vi "Finish.vi"   [LabVIEW 2013]
doc: "This VI is called just before exiting. It is expected to close I/O refnum, save collected data, etc."
uses:
  <vilib>/Rock Robotics/WPI/Joystick/WPI_JoystickGetSetRefNum.vi
  <vilib>/Rock Robotics/WPI/RobotDrive/WPI_RobotDriveGetSetRefNum.vi
types:
  T1 = typedef "WPI_JoystickDevRef.ctl" = cluster{"Device":T2}
  T2 = typedef "WPI_JoystickDeviceEnum.ctl" = enum16{"USB 1", "USB 2", "USB 3", "USB 4", "Kinect 1", "Kinect 2"}
  T3 = typedef "WPI_RobotDriveDevRef.ctl" = cluster{"DevStatus":errorcluster, "Motors[]":T4[], "Square Inputs":bool, "Max Output":dbl, "Isochronous":bool}
  T4 = typedef "WPI_MotorControlDeviceRef.ctl" = cluster{"DeviceStatus":errorcluster, "Type":enum16{"PWM", "CAN"}, "PWM":cluster{"Digital Module":T5, "PWM Channel":T6, "DeadBand":T7}, "CAN":cluster{"Device Number":u8, "Control Mode":T8, "Semaphore":T9, "Max Vout":dbl}, "Invert":bool, "TransformRef":T10, "InvTransformRef":T10}
  T5 = typedef "FPGA_TypedefDigitalModule.ctl" = enum16{"Digital Module 1", "Digital Module 2"}
  T6 = typedef "FPGA_DIOPWMChannel.ctl" = enum8{"PWM 1", "PWM 2", "PWM 3", "PWM 4", "PWM 5", "PWM 6", "PWM 7", "PWM 8", "PWM 9", "PWM 10", "Invalid"}
  T7 = typedef "WPI_PWMDeadband.ctl" = cluster{"Name":string, "maxPositivePwm":i32, "minPositivePwm":i32, "centerPwm":i32, "maxNegativePwm":i32, "minNegativePwm":i32, "angularRange":u16}
  T8 = typedef "WPI_CANJaguar_ControlMode.ctl" = enum8{"Percent VBus", "Current", "Speed", "Position", "Voltage"}
  T9 = typedef "Semaphore RefNum" = refnum<k1>
  T10 = typedef "WPI_PWMTransform_ConPane.ctl" = refnum<vi>
  T11 = typedef "WPI_GyroDevRef.ctl" = cluster{"DevStatus":errorcluster, "Analog Module":T12, "Analog Channel":T13, "Offset":dbl, "Gain (VoltsPerDegree/Second)":dbl}
  T12 = typedef "FPGA_TypedefAnalogModule.ctl" = enum16{"Analog Module 1", "Analog Module 2"}
  T13 = typedef "FPGA_AIChannel.ctl" = enum8{"AI 1", "AI 2", "AI 3", "AI 4", "AI 5", "AI 6", "AI 7", "AI 8", "Invalid"}
  T14 = typedef "WPI_EncoderDevRef.ctl" = cluster{"DevStatus":errorcluster, "EncoderIndex":T15, "CounterIndex":T16, "DistancePerCount":dbl, "Decoding Type":T17}
  T15 = typedef "FPGA_EncoderIdx.ctl" = enum8{"Enc 0", "Enc 1", "Enc 2", "Enc 3", "Invalid"}
  T16 = typedef "FPGA_CounterCtrSystemIndex.ctl" = enum8{"Ctr 0", "Ctr 1", "Ctr 2", "Ctr 3", "Ctr 4", "Ctr 5", "Ctr 6", "Ctr 7", "Invalid"}
  T17 = typedef "WPI_EncoderType.ctl" = enum16{"1x", "2x", "4x"}
  T18 = cluster{"Motors[]":T14[], "DevStatus":errorcluster, "Max Speed[]":dbl[]}
  T19 = typedef "WPI_RelayDevRef.ctl" = cluster{"DevStatus":errorcluster, "Relay Channel":T20, "Digital Module":T5, "Relay Direction":T21}
  T20 = typedef "FPGA_DIORelayChannel.ctl" = enum8{"Relay 1", "Relay 2", "Relay 3", "Relay 4", "Relay 5", "Relay 6", "Relay 7", "Relay 8", "Invalid"}
  T21 = typedef "WPI_RelayDirection.ctl" = enum16{"Both directions", "Forward only", "Reverse only"}
  T22 = typedef "WPI_SolenoidDevRef.ctl" = cluster{"DevStatus":errorcluster, "Solenoid Module":T23, "Forward Solenoid Channel":T24, "Reverse Solenoid Channel":T24}
  T23 = typedef "FPGA_TypedefSolenoidModule.ctl" = enum16{"Solenoid Module 1", "Solenoid Module 2"}
  T24 = typedef "WPI_SolenoidChannel.ctl" = enum8{"Solenoid 1", "Solenoid 2", "Solenoid 3", "Solenoid 4", "Solenoid 5", "Solenoid 6", "Solenoid 7", "Solenoid 8", "Invalid"}
  T25 = typedef "WPI_AnalogChannelDevRef.ctl" = cluster{"DevStatus":errorcluster, "Analog Module":T12, "Analog Channel":T13}
  T26 = typedef "WPI_I2CDevRef.ctl" = cluster{"DevStatus":errorcluster, "Digital Module":T5, "Device Address":u8}
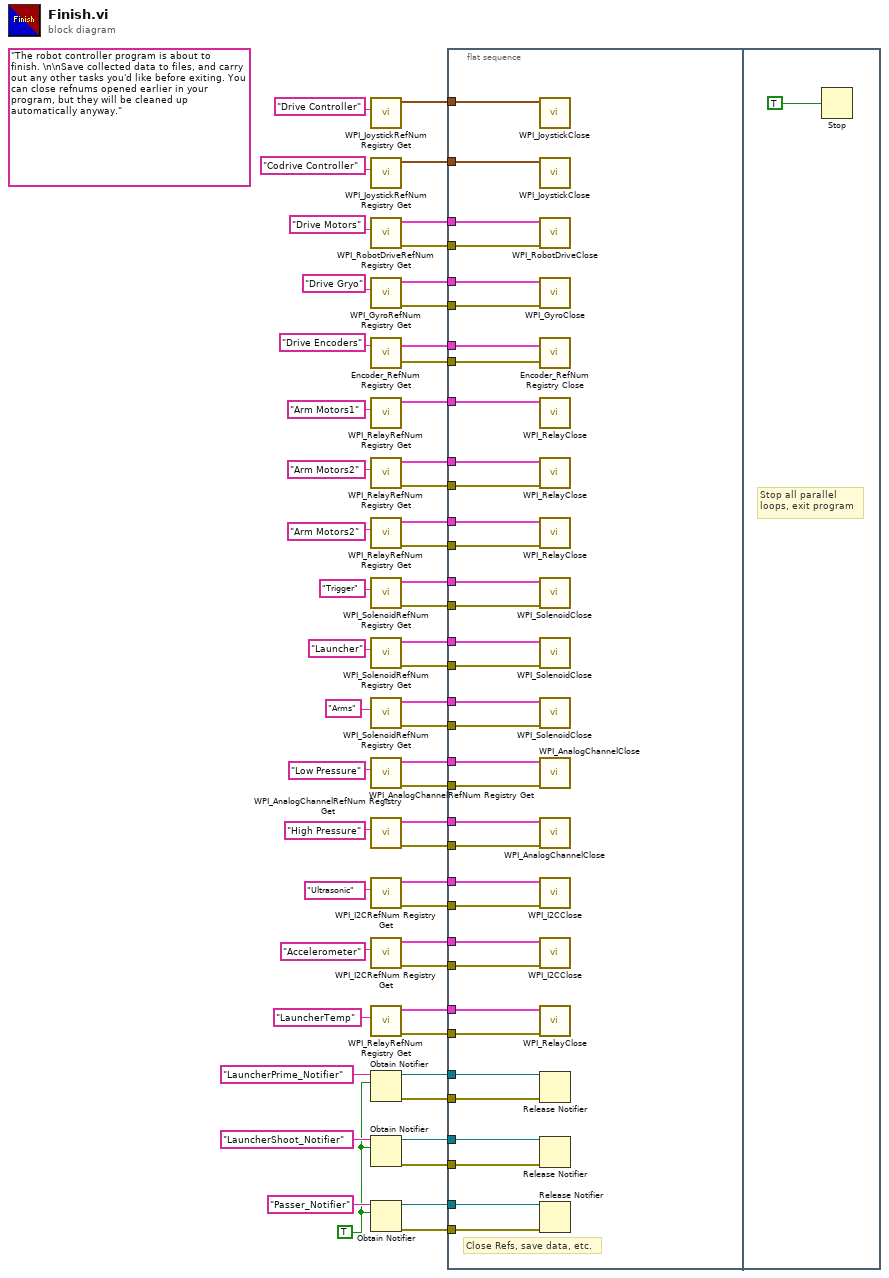
[diagram p0: block diagram]
diagram:
  w1 = TRUE
  (unwired) "The robot controller program is about to finish. \n\nSave collected data to files, and carry out any other tasks you'd like before exiting. You can close refnums opened earlier in your program, but they will be cleaned up automatically anyway."
  n1 = call <vilib>:"WPI_JoystickRefNum Registry Get.vi"("refnum name"="Drive Controller") -> ("JoystickDevRef"=w52:T1)  [unwired: 1 in, 9 out]
  n2 = call <vilib>:"WPI_JoystickRefNum Registry Get.vi"("refnum name"="Codrive Controller") -> ("JoystickDevRef"=w39:T1)  [unwired: 1 in, 9 out]
  n3 = call <vilib>:"WPI_RobotDriveRefNum Registry Get.vi"("refnum name"="Drive Motors") -> ("error out"=w49:errorcluster, "RobotDriveDevRef"=w53:T3)  [unwired: 1 in, 8 out]
  n4 = call <vilib>:"WPI_GyroRefNum Registry Get.vi"("refnum name"="Drive Gryo") -> ("error out"=w50:errorcluster, "GyroDevRef"=w51:T11)  [unwired: 9 in]
  n5 = call "Encoder_RefNum Registry Get.vi"("refnum name"="Drive Encoders") -> ("error out"=w45:errorcluster, "RobotEncoderRef Out"=w46:T18)  [unwired: 1 in]
  n6 = call <vilib>:"WPI_RelayRefNum Registry Get.vi"("refnum name"="Arm Motors1") -> ("RelayDevRef"=w38:T19)  [unwired: 9 in, 1 out]
  n7 = call <vilib>:"WPI_RelayRefNum Registry Get.vi"("refnum name"="Arm Motors2") -> ("error out"=w36:errorcluster, "RelayDevRef"=w37:T19)  [unwired: 9 in]
  n8 = call <vilib>:"WPI_RelayRefNum Registry Get.vi"("refnum name"="Arm Motors2") -> ("error out"=w15:errorcluster, "RelayDevRef"=w14:T19)  [unwired: 9 in]
  n9 = call <vilib>:"WPI_SolenoidRefNum Registry Get.vi"("refnum name"="Trigger") -> ("error out"=w31:errorcluster, "SolenoidDevRef"=w33:T22)  [unwired: 9 in]
  n10 = call <vilib>:"WPI_SolenoidRefNum Registry Get.vi"("refnum name"="Launcher") -> ("error out"=w30:errorcluster, "SolenoidDevRef"=w32:T22)  [unwired: 9 in]
  n11 = call <vilib>:"WPI_SolenoidRefNum Registry Get.vi"("refnum name"="Arms") -> ("error out"=w18:errorcluster, "SolenoidDevRef"=w19:T22)  [unwired: 9 in]
  n12 = call <vilib>:"WPI_AnalogChannelRefNum Registry Get.vi"("refnum name"="Low Pressure") -> ("error out"=w23:errorcluster, "AIDeviceRef"=w25:T25)  [unwired: 9 in]
  n13 = call <vilib>:"WPI_AnalogChannelRefNum Registry Get.vi"("refnum name"="High Pressure") -> ("error out"=w22:errorcluster, "AIDeviceRef"=w24:T25)  [unwired: 9 in]
  n14 = call <vilib>:"WPI_I2CRefNum Registry Get.vi"("refnum name"="Ultrasonic") -> ("error out"=w43:errorcluster, "I2CDevRef"=w44:T26)  [unwired: 9 in]
  n15 = call <vilib>:"WPI_I2CRefNum Registry Get.vi"("refnum name"="Accelerometer") -> ("error out"=w41:errorcluster, "I2CDevRef"=w42:T26)  [unwired: 9 in]
  n16 = call <vilib>:"WPI_RelayRefNum Registry Get.vi"("refnum name"="LauncherTemp") -> ("error out"=w12:errorcluster, "RelayDevRef"=w13:T19)  [unwired: 9 in]
  n17 = Obtain Notifier(name (unnamed)="LauncherPrime_Notifier", notification data type=w1) -> (notifier out=w10:refnum<notifier>, error out=w5:errorcluster)  [unwired: 2 in, 1 out]
  n18 = Obtain Notifier(name (unnamed)="LauncherShoot_Notifier", notification data type=w1) -> (notifier out=w9:refnum<notifier>, error out=w8:errorcluster)  [unwired: 2 in, 1 out]
  n19 = Obtain Notifier(name (unnamed)="Passer_Notifier", notification data type=w1) -> (notifier out=w7:refnum<notifier>, error out=w6:errorcluster)  [unwired: 2 in, 1 out]
  n20 = flat-sequence {
    tunnel: w53 -> [w90]
    tunnel: w52 -> [w89]
    tunnel: w51 -> [w88]
    tunnel: w50 -> [w87]
    tunnel: w49 -> [w86]
    tunnel: w46 -> [w85]
    tunnel: w45 -> [w84]
    tunnel: w44 -> [w83]
    tunnel: w43 -> [w82]
    tunnel: w42 -> [w81]
    tunnel: w41 -> [w80]
    tunnel: w39 -> [w79]
    tunnel: w38 -> [w78]
    tunnel: w37 -> [w77]
    tunnel: w36 -> [w76]
    tunnel: w33 -> [w75]
    tunnel: w32 -> [w74]
    tunnel: w31 -> [w73]
    tunnel: w30 -> [w72]
    tunnel: w25 -> [w71]
    tunnel: w24 -> [w70]
    tunnel: w23 -> [w69]
    tunnel: w22 -> [w68]
    tunnel: w19 -> [w67]
    tunnel: w18 -> [w66]
    tunnel: w15 -> [w64]
    tunnel: w14 -> [w65]
    tunnel: w13 -> [w63]
    tunnel: w12 -> [w62]
    tunnel: w10 -> [w61]
    tunnel: w9 -> [w60]
    tunnel: w8 -> [w59]
    tunnel: w7 -> [w58]
    tunnel: w6 -> [w57]
    tunnel: w5 -> [w56]
    frame #0 {
      # "Close Refs, save data, etc."
      n21 = call <vilib>:"WPI_JoystickClose.vi"("JoystickDevRef"=w89) -> ()  [unwired: 11 out]
      n22 = call <vilib>:"WPI_JoystickClose.vi"("JoystickDevRef"=w79) -> ()  [unwired: 11 out]
      n23 = call <vilib>:"WPI_RobotDriveClose.vi"("error in (no error)"=w86, "RobotDriveDevRef"=w90) -> ()  [unwired: 10 out]
      n24 = call <vilib>:"WPI_GyroClose.vi"("error in (no error)"=w87, "GyroDevRef"=w88) -> ()  [unwired: 9 in, 1 out]
      n25 = call "Encoder_RefNum Registry Close.vi"("error in (no error)"=w84, "RobotEncoderRef"=w85) -> ()  [unwired: 1 out]
      n26 = call <vilib>:"WPI_RelayClose.vi"("RelayDevRef"=w78) -> ()  [unwired: 10 in, 1 out]
      n27 = call <vilib>:"WPI_RelayClose.vi"("error in (no error)"=w76, "RelayDevRef"=w77) -> ()  [unwired: 9 in, 1 out]
      n28 = call <vilib>:"WPI_RelayClose.vi"("error in (no error)"=w64, "RelayDevRef"=w65) -> ()  [unwired: 9 in, 1 out]
      n29 = call <vilib>:"WPI_SolenoidClose.vi"("error in (no error)"=w73, "SolenoidDevRef"=w75) -> ()  [unwired: 9 in, 1 out]
      n30 = call <vilib>:"WPI_SolenoidClose.vi"("error in (no error)"=w72, "SolenoidDevRef"=w74) -> ()  [unwired: 9 in, 1 out]
      n31 = call <vilib>:"WPI_SolenoidClose.vi"("error in (no error)"=w66, "SolenoidDevRef"=w67) -> ()  [unwired: 9 in, 1 out]
      n32 = call <vilib>:"WPI_AnalogChannelClose.vi"("error in (no error)"=w69, "AIDeviceRef"=w71) -> ()  [unwired: 9 in, 1 out]
      n33 = call <vilib>:"WPI_AnalogChannelClose.vi"("error in (no error)"=w68, "AIDeviceRef"=w70) -> ()  [unwired: 9 in, 1 out]
      n34 = call <vilib>:"WPI_I2CClose.vi"("error in (no error)"=w82, "I2CDevRef"=w83) -> ()  [unwired: 9 in, 1 out]
      n35 = call <vilib>:"WPI_I2CClose.vi"("error in (no error)"=w80, "I2CDevRef"=w81) -> ()  [unwired: 9 in, 1 out]
      n36 = call <vilib>:"WPI_RelayClose.vi"("error in (no error)"=w62, "RelayDevRef"=w63) -> ()  [unwired: 9 in, 1 out]
      n37 = Release Notifier(notifier=w61, error in (no error)=w56) -> ()  [unwired: 1 in, 3 out]
      n38 = Release Notifier(notifier=w60, error in (no error)=w59) -> ()  [unwired: 1 in, 3 out]
      n39 = Release Notifier(notifier=w58, error in (no error)=w57) -> ()  [unwired: 1 in, 3 out]
    }
    frame #1 {
      # "Stop all parallel\nloops, exit program"
      n40 = Stop(stop? (T)=TRUE ("Quit")) -> ()
    }
  }
